vi "forward power dBm subvi.vi"(3 "error in (no error)":errorcluster, 5 "VISA resource name":refnum<visa-resource-name>="GPIB0::12::INSTR") -> (0 "error out":errorcluster, 1 "forward power (dBm)":dbl, 2 "VISA resource name out":refnum<visa-resource-name>)   [LabVIEW 2009]
panel:
  out "read buffer":string
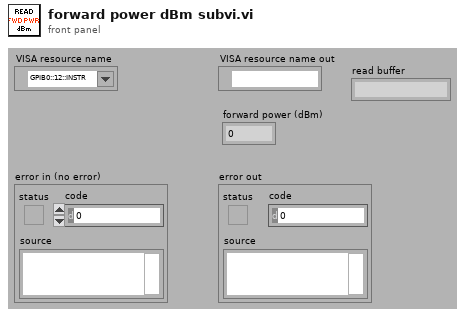
[diagram p1: front panel]
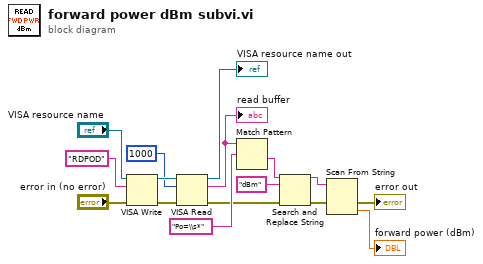
[diagram p0: block diagram]
diagram:
  n1 = VISA Write(VISA resource name="VISA resource name", write buffer="RDPOD", error in (no error)="error in (no error)") -> (VISA resource name out=w15:refnum<visa-resource-name>, error out=w14:errorcluster)  [unwired: 1 out]
  n2 = VISA Read(VISA resource name=w15, byte count=u32 1000 ("bytes to read (1000)"), error in (no error)=w14) -> (VISA resource name out=→"VISA resource name out":refnum<visa-resource-name>, read buffer=w8:string, error out=w3:errorcluster)  [unwired: 1 out]
  "read buffer" <- w8
  n3 = Match Pattern(string=w8, regular expression="Po=\\s*" ("search string")) -> (after substring=w6:string)  [unwired: 1 in, 3 out]
  n4 = Search and Replace String(input string=w6, search string="dBm", error in=w3) -> (result string=w5:string, error out=w2:errorcluster)  [unwired: 5 in, 2 out]
  n5 = Scan From String(input string=w5, error in=w2) -> (error out=→"error out":errorcluster, output 1=→"forward power (dBm)":dbl)  [unwired: 3 in, 2 out]
